vi "Frequency to motor position.vi"(10 "Fit parameters":cluster{"Slope":dbl, "Intercept":dbl}, 11 "Frequency":dbl) -> (3 "Motor position":dbl)   [LabVIEW 2015]
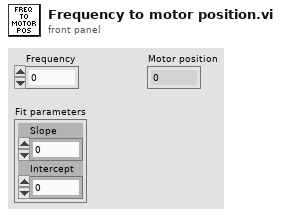
[diagram p1: front panel]
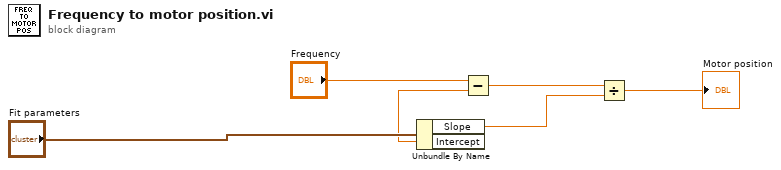
[diagram p0: block diagram]
diagram:
  n1 = Unbundle By Name("Fit parameters") -> ("Slope"=w5:dbl, "Intercept"=w4:dbl)
  n2 = Subtract(x="Frequency", y=w4) -> (x-y=w1:dbl)
  n3 = Divide(x=w1, y=w5) -> (x/y=→"Motor position":dbl)
